vi "main-6003.vi"() -> ()   [LabVIEW 2018]
uses:
  <vilib>/Utility/miscctls.llb/LVPointDoubleTypeDef.ctl
  <vilib>/DAQmx/read.llb/DAQmx Read (Analog 1D Wfm NChan NSamp).vi
  <vilib>/Analysis/baseanly.llb/Mean (DBL).vi
  <vilib>/DAQmx/create/channels.llb/DAQmx Create Channel (AI-Voltage-Basic).vi
  <vilib>/DAQmx/configure/timing.llb/DAQmx Timing (Sample Clock).vi
  <vilib>/DAQmx/miscellaneous.llb/DAQmx Fill In Error Info.vi
  <vilib>/Waveform/WDTOps.llb/WDT Append Waveforms DBL.vi
  <vilib>/Utility/file.llb/Write To Spreadsheet File (DBL).vi
  <vilib>/Analysis/NI_AALBase.lvlib
  <resource>/objmgr/daqmx.rc
panel:
  out "当前":dbl
  in  "label":string
  out "时序":waveform(dbl)[](graph)
  out "判断类型":dbl
  out "可能性":dbl
  out "不同物品相似值":dbl[](graph)
  in  "?":bool
  in  "AIConv.Rate":dbl=5001.0
  in  "Channel":i32=1 min=1 max=6 step=1
  out "数组":string[](array[string])
  in  "选项卡控件":enum32{"Multichannel", "Single Channel"}(tab)
  out "Resistance":waveform(dbl)[](graph)
  out "Voltage":waveform(dbl)[](graph)
  in  "下拉列表 2":u16(ring) items=["Linear", "Log"]
  in  "Cursor":bool
  in  "下拉列表":u16(ring) items=["Linear", "Log"]
  in  "Cursor":bool
  out "游标.游标位置 2":T1 caption="游标.游标位置" {"Y" format="%#_5g"}
  out "游标.游标位置":T1
  out "游标.游标位置 4":T1 caption="游标.游标位置" {"Y" format="%#_5g"}
  in  "下拉列表 5":u16(ring) items=["Linear", "Log"]
  in  "Cursor":bool
  in  "下拉列表 4":u16(ring) items=["Linear", "Log"]
  in  "Cursor":bool
  out "Resistance":waveform(dbl)(graph)
  out "Voltage":waveform(dbl)(graph)
  out "游标.游标位置 3":T1 caption="游标.游标位置" {"Y" format="%#_5g"}
  out "元素 2":dbl format="%#_5g"
  out "元素":dbl format="%#_5p"
  in  "Resistance":dbl=100000.0
  in  "channel":i32=6 min=1 max=10 step=1
  in  "Voltage":dbl=1.0 min=-10.0 max=10.0
  out "default":path
  out "Elapsed Time (s)":dbl caption="Elapse Time"
  in  "确定按钮 2":bool
  in  "停止 2":bool
  in  "确定按钮":bool
  in  "停止":bool
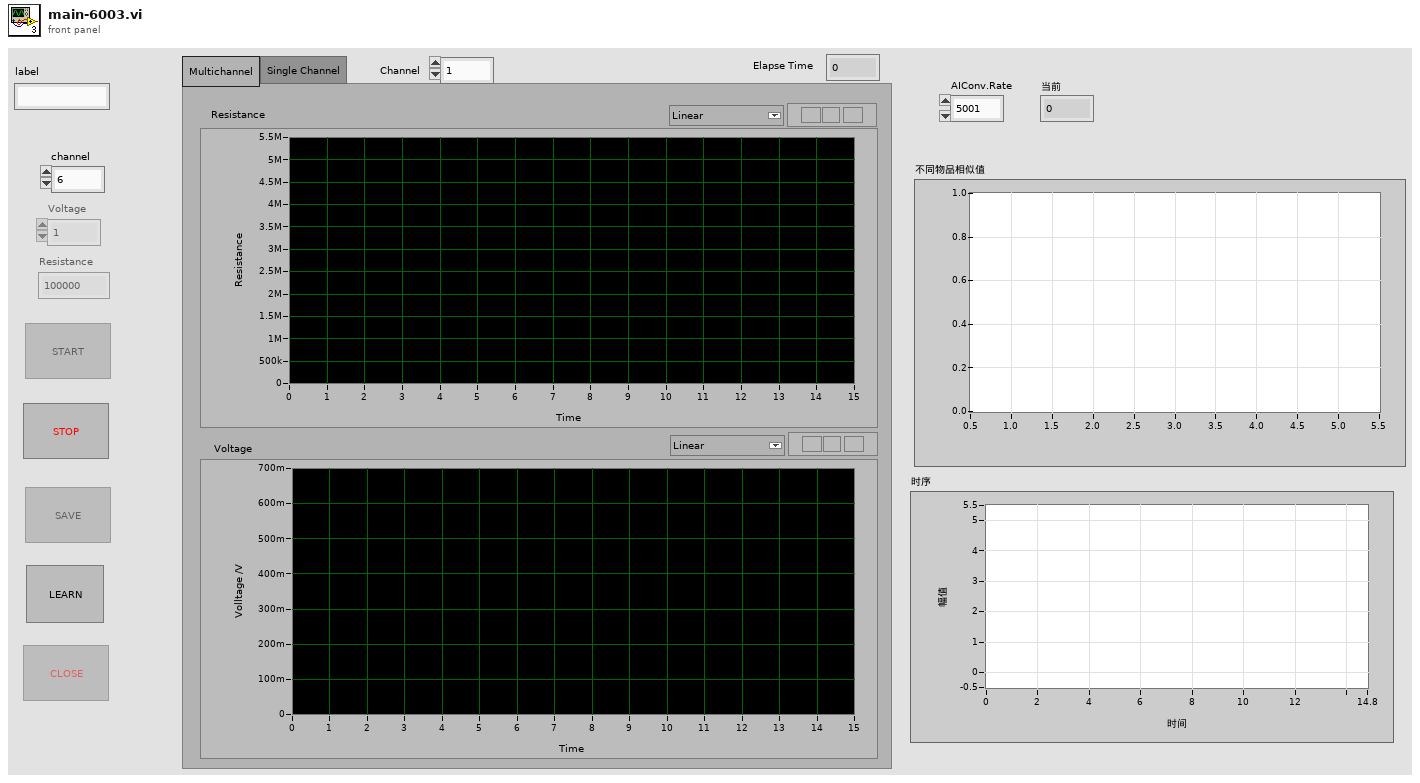
[diagram p1: front panel]
types:
  T1 = typedef "LVPointDoubleTypeDef.ctl" = cluster{"X":dbl, "Y":dbl}
  T2 = enum8{"Enabled", "Disabled", "Disabled and Grayed Out"}
  T3 = enum32{"invalid app kind", "Development System", "Run Time System", "Student Edition", "Embedded LabVIEW", "Evaluation", "Custom"}
  T4 = typedef "LVAnnotationListTypeDef.ctl" = cluster{"Name":string, "Color":u32, "Style":u8, "Point Style":u8, "Name Visible":bool, "Allow Drag":bool, "Annotation Mode":u32, "Plot":i32, "Index":i32, "Position":cluster{"X":dbl, "Y":dbl}, "X Scale":u32, "Y Scale":u32, "Show Arrow":bool, "Lock Name":bool, "Plot Area":i32, "Label Offset":cluster{"X":dbl, "Y":dbl}}[]
  T5 = cluster{"Name":string, "Color":u32, "Style":u8, "Point Style":u8, "Name Visible":bool, "Allow Drag":bool, "Annotation Mode":u32, "Plot":i32, "Index":i32, "Position":cluster{"X":dbl, "Y":dbl}, "X Scale":u32, "Y Scale":u32, "Show Arrow":bool, "Lock Name":bool, "Plot Area":i32, "Label Offset":cluster{"X":dbl, "Y":dbl}}
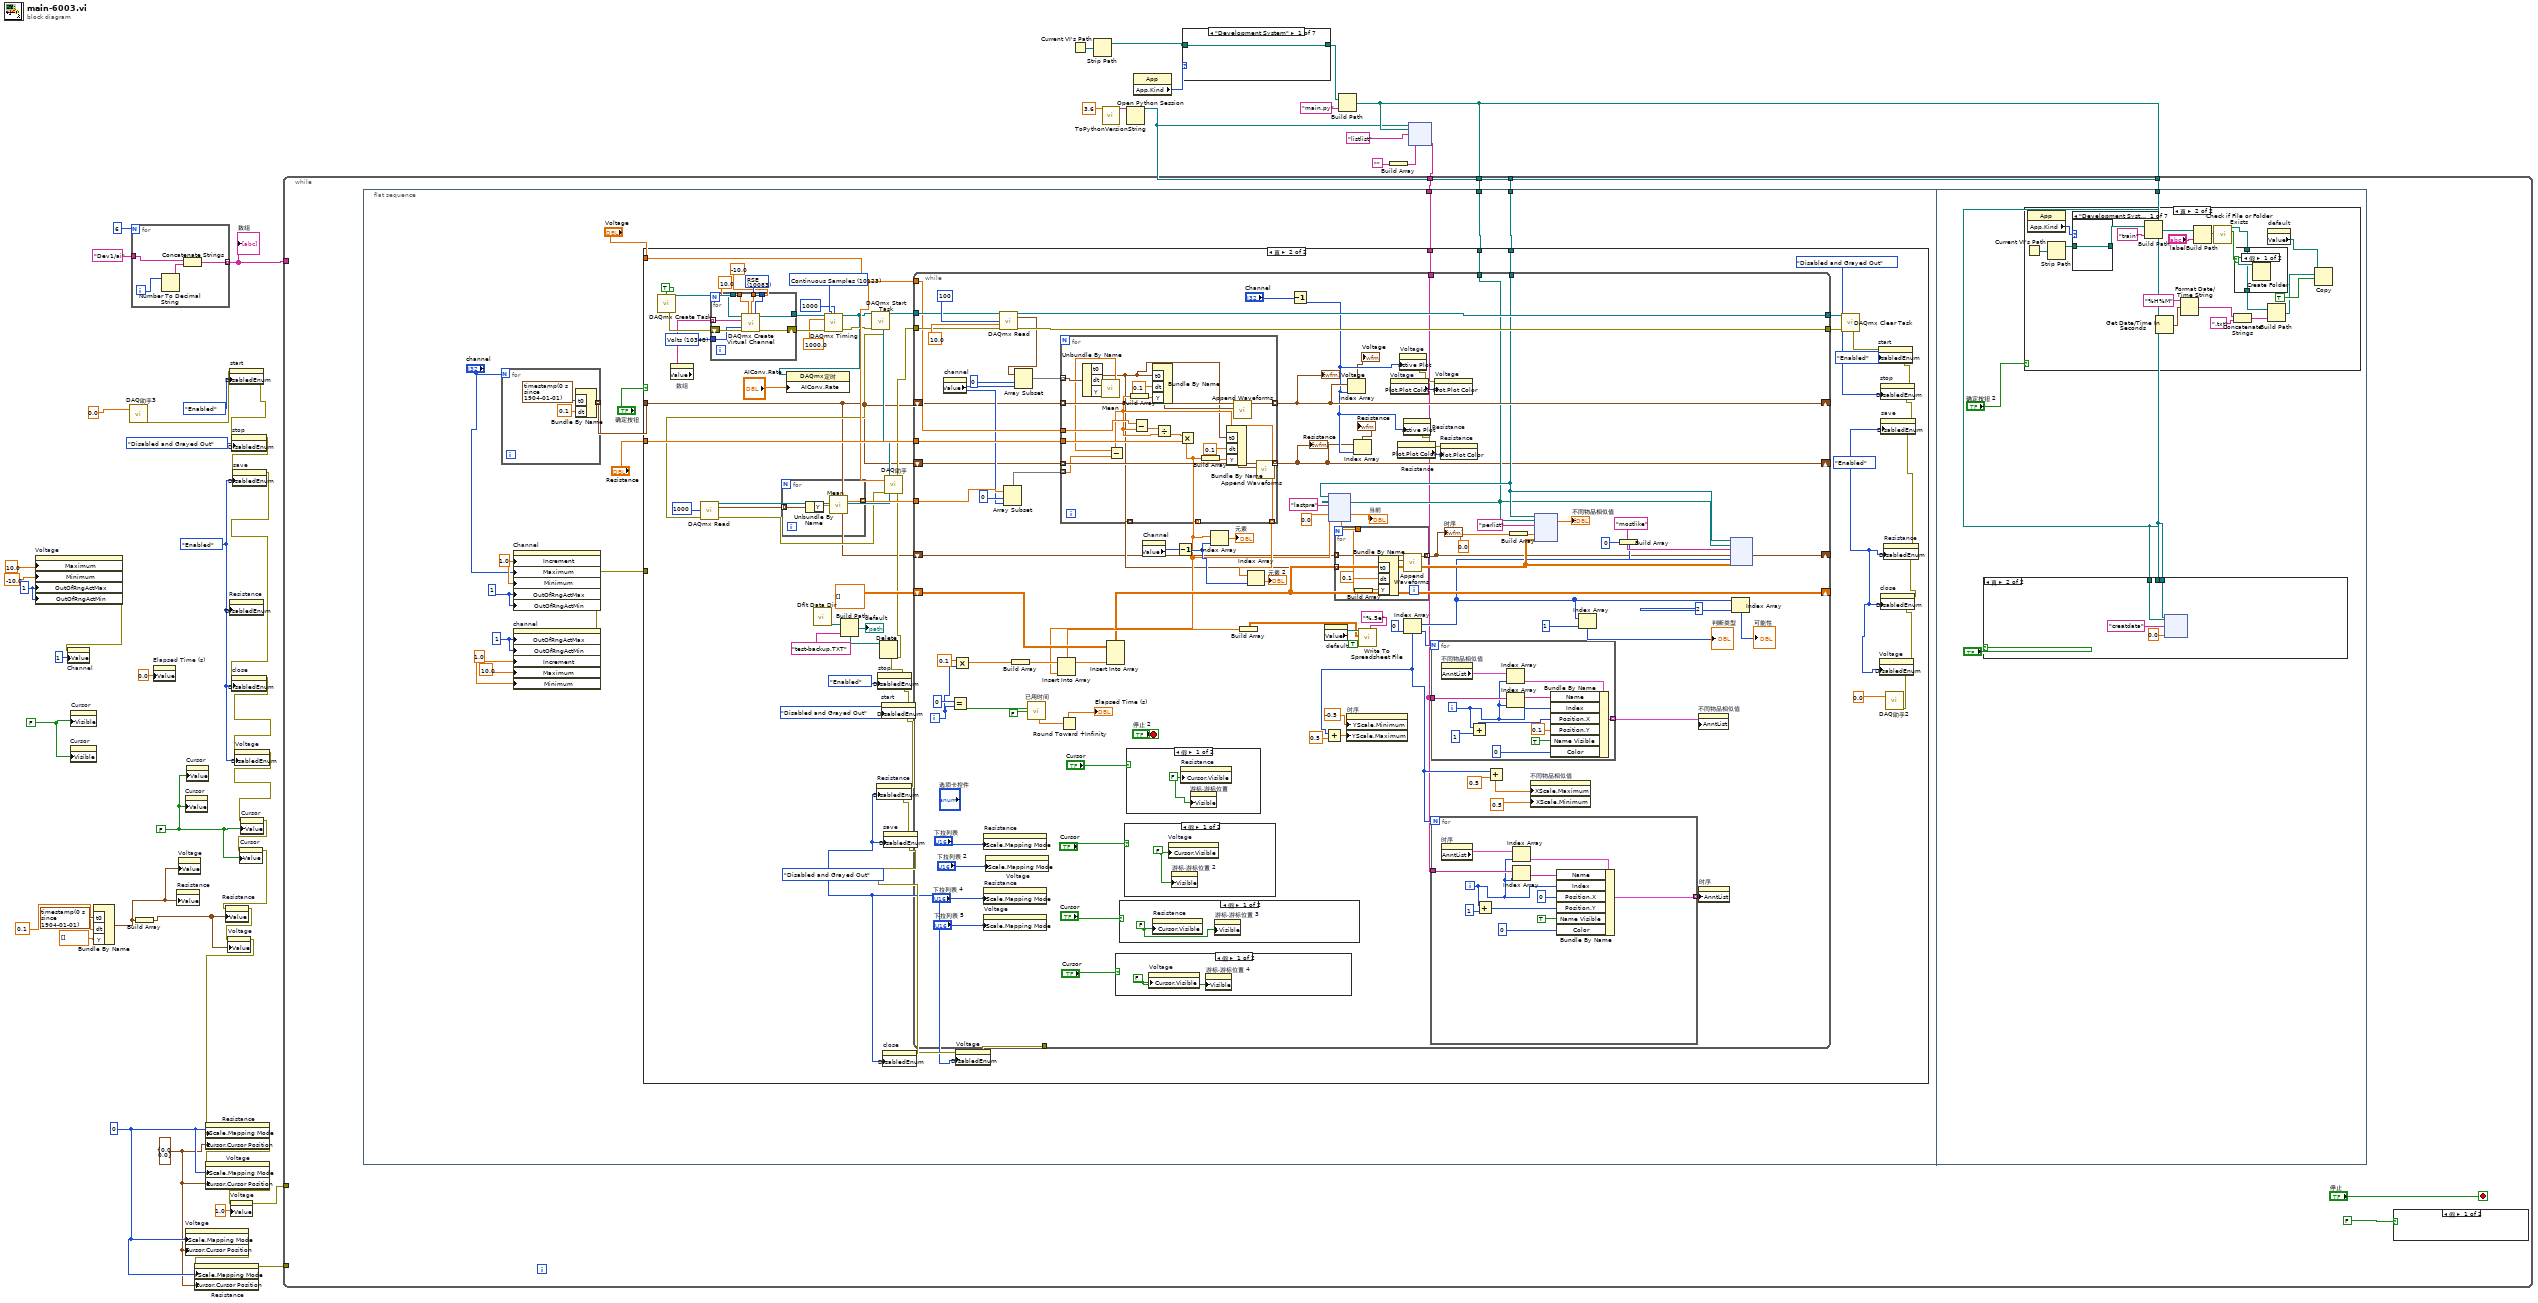
[diagram p0: block diagram]
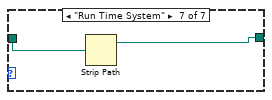
[diagram p7: hidden frame]
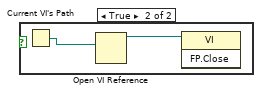
[diagram p8: hidden frame]
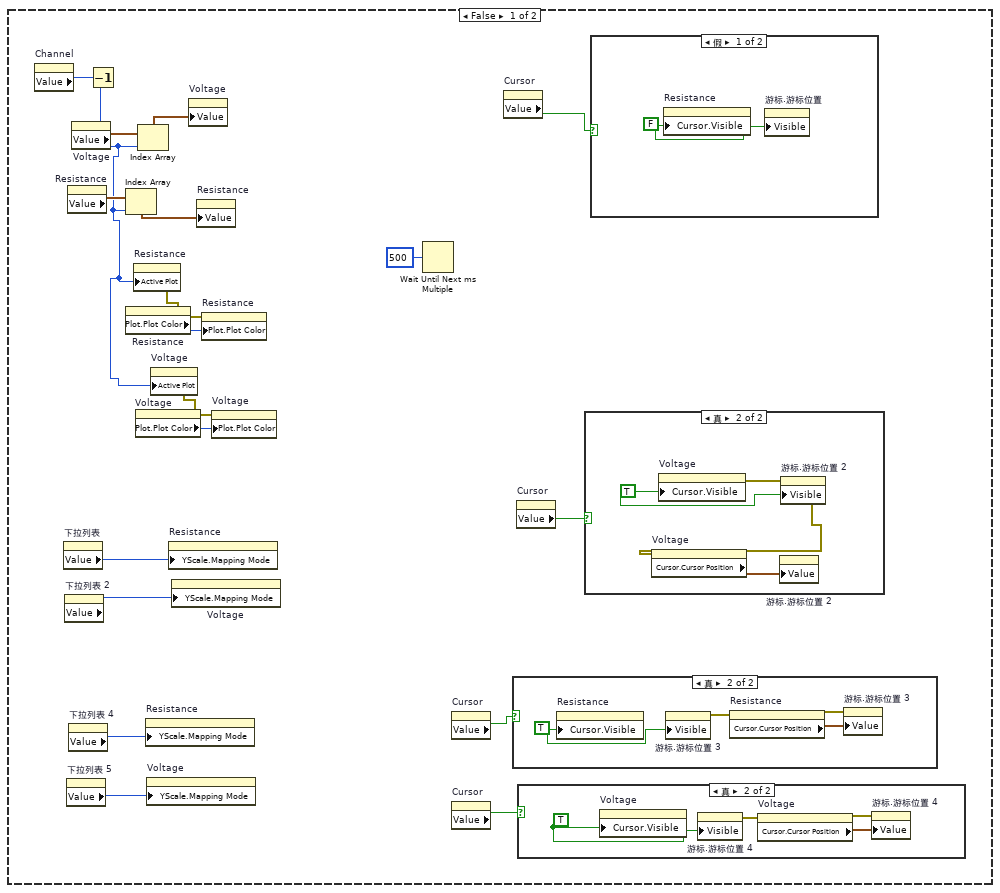
[diagram p9: hidden frame]
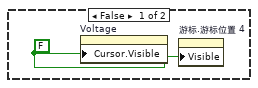
[diagram p10: hidden frame]
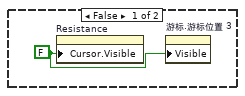
[diagram p11: hidden frame]
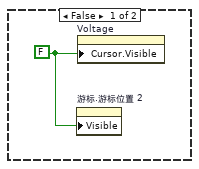
[diagram p12: hidden frame]
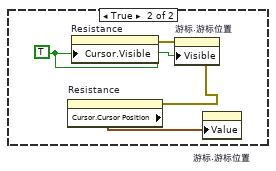
[diagram p13: hidden frame]
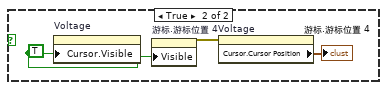
[diagram p14: hidden frame]
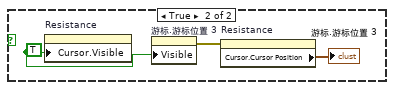
[diagram p15: hidden frame]
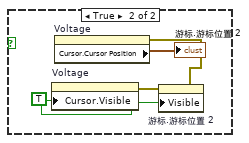
[diagram p16: hidden frame]
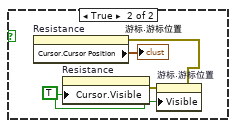
[diagram p17: hidden frame]
diagram:
  w19 = u8 1 ("对超出界限的值的响应:最大值")
  w28 = FALSE ("可见")
  w26 = FALSE ("Cursor")
  w24 = T1 {"X"=0.0, "Y"=0.0} ("游标.游标位置")
  w25 = u8 0 ("Y标尺.映射模式")
  w17 = T2."Enabled" ("禁用")
  n1 = property on="Voltage" class="DigNum (严格)"("Maximum"=10.0 ("数据输入界限:最大值"), "Minimum"=-10.0 ("数据输入界限:最大值"), "OutOfRngActMax"=w19, "OutOfRngActMin"=w19) -> (error out=w20:errorcluster)  [unwired: 2 in, 1 out]
  n2 = property on="Channel" class="DigNum (严格)"(error in=w20, "Value"=1 ("index (row)")) -> ()  [unwired: 1 in, 2 out]
  n3 = property on="Cursor" class="Bool (严格)"("Visible"=w28) -> ()  [unwired: 2 in, 2 out]
  n4 = property on="Cursor" class="Bool (严格)"("Visible"=w28) -> ()  [unwired: 2 in, 2 out]
  n5 = Bundle By Name("t0"=timestamp(0 s since 1904-01-01), "dt"=0.1, "Y"=dbl[] []) -> (w27:waveform(dbl))  [unwired: 1 in]
  n6 = call "DAQ助手3"("data"=0.0 ("maximum value")) -> ("error out"=w30:errorcluster)  [unwired: 17 in, 1 out]
  n7 = for {
    N: 6 -> [_]
    tunnel: "Dev1/ai" -> [w54]
    tunnel: [w52] -> w18 mode=indexing
    i -> [w55]
    n8 = Number To Decimal String(number=w55) -> (decimal integer string=w53:string)  [unwired: 1 in]
    n9 = Concatenate Strings(w54, w53) -> (w52:string)
  }
  "数组" <- w18
  n10 = Build Array(w27) -> (w32:waveform(dbl)[])
  n11 = property on="Elapsed Time (s)" class="DigNum (严格)"("Value"=0.0 ("Elapsed Time (s)")) -> ()  [unwired: 2 in, 2 out]
  n12 = property on="Resistance" class="WFGraph (严格)"("Value"=w27) -> ()  [unwired: 2 in, 2 out]
  n13 = property on="Voltage" class="WFGraph (严格)"("Value"=w27) -> ()  [unwired: 2 in, 2 out]
  n14 = property on="Cursor" class="Bool (严格)"("Value"=w26) -> ()  [unwired: 2 in, 2 out]
  n15 = property on="Voltage" class="WFGraph (严格)"("YScale.Mapping Mode"=w25, "Cursor.Cursor Position"=w24) -> (error out=w15:errorcluster)  [unwired: 2 in, 1 out]
  n16 = property on="Cursor" class="Bool (严格)"("Value"=w26) -> ()  [unwired: 2 in, 2 out]
  n17 = property on="Resistance" class="WFGraph (严格)"(error in=w15, "YScale.Mapping Mode"=w25, "Cursor.Cursor Position"=w24) -> (error out=w16:errorcluster)  [unwired: 1 in, 1 out]
  n18 = property on="Resistance" class="DigNum (严格)"("DisabledEnum"=w17) -> ()  [unwired: 2 in, 2 out]
  n19 = property on="start" class="Bool"(error in=w30, "DisabledEnum"=T2."Enabled" ("禁用")) -> (error out=w49:errorcluster)  [unwired: 1 in, 1 out]
  n20 = property on="stop" class="Bool"(error in=w49, "DisabledEnum"=T2."Disabled and Grayed Out" ("禁用")) -> (error out=w48:errorcluster)  [unwired: 1 in, 1 out]
  n21 = property on="save" class="Bool"(error in=w48, "DisabledEnum"=w17) -> (error out=w39:errorcluster)  [unwired: 1 in, 1 out]
  n22 = property on="close" class="Bool"(error in=w39, "DisabledEnum"=w17) -> (error out=w38:errorcluster)  [unwired: 1 in, 1 out]
  n23 = property on="Voltage" class="DigNum (严格)"(error in=w38, "DisabledEnum"=w17) -> (error out=w37:errorcluster)  [unwired: 1 in, 1 out]
  n24 = property on="Cursor" class="Bool (严格)"(error in=w37, "Value"=w26) -> (error out=w42:errorcluster)  [unwired: 1 in, 1 out]
  n25 = property on="Cursor" class="Bool (严格)"(error in=w42, "Value"=w26) -> (error out=w41:errorcluster)  [unwired: 1 in, 1 out]
  n26 = property on="Resistance" class="WFGraph (严格)"(error in=w41, "Value"=w32) -> (error out=w47:errorcluster)  [unwired: 1 in, 1 out]
  n27 = property on="Voltage" class="WFGraph (严格)"(error in=w47, "Value"=w32) -> (error out=w46:errorcluster)  [unwired: 1 in, 1 out]
  n28 = property on="Resistance" class="WFGraph (严格)"(error in=w46, "YScale.Mapping Mode"=w25, "Cursor.Cursor Position"=w24) -> (error out=w45:errorcluster)  [unwired: 1 in, 1 out]
  n29 = property on="Voltage" class="WFGraph (严格)"(error in=w45, "YScale.Mapping Mode"=w25, "Cursor.Cursor Position"=w24) -> (error out=w44:errorcluster)  [unwired: 1 in, 1 out]
  n30 = property on="Voltage" class="DigNum (严格)"(error in=w44, "Value"=1.0 ("Voltage")) -> (error out=w36:errorcluster)  [unwired: 1 in, 1 out]
  n31 = Current VI's Path() -> (path=w10:path)
  n32 = Strip Path(path=w10) -> (stripped path=w2:path)  [unwired: 1 out]
  n33 = call "ToPythonVersionString.vi"("Python版本"=3.6) -> ("python版本字符串"=w12:string)  [unwired: 10 in]
  n34 = Open Python Session(python version=w12) -> (session out=w4:refnum<k35>)  [unwired: 2 in, 1 out]
  n35 = property class="App"() -> ("App.Kind"=w3:T3)  [unwired: 2 in, 2 out]
  n36 = case shown="\"Development System\"" w3 {
    tunnel: w2 -> [w56 w57 w58 w59 w60 w61 w63]
    tunnel: [w56 w57 w58 w59 w60 w61 w62] -> w1
    frame "Development System" {
    }
    frame "Embedded LabVIEW" {
    }
    frame "Student Edition" {
    }
    frame "invalid app kind" {
    }
    frame "Custom" {
    }
    frame "Evaluation" {
    }
    frame "Run Time System" {
      n37 = Strip Path(path=w63) -> (stripped path=w62:path)  [unwired: 1 out]
    }
  }
  n38 = Build Path(base path=w1, name or relative path="main.py") -> (appended path=w5:path)
  n39 = Build Array("") -> (w7:string[])
  n40 = node(w4, w5, "listlist", w7) -> (w6:string[])  [unwired: 1 in, 4 out]
  n41 = while {
    tunnel: w36 -> [_]
    tunnel: w18 -> [_]
    tunnel: w16 -> [_]
    tunnel: w4 -> [w68]
    tunnel: w5 -> [w67]
    tunnel: w6 -> [w66]
    tunnel: w5 -> [w65]
    tunnel: w4 -> [w64]
    stop <- "停止" stop-if-true
    n42 = flat-sequence {
      tunnel: w66 -> [w75]
      tunnel: w65 -> [w74]
      tunnel: w64 -> [w73]
      tunnel: w68 -> [w360]
      tunnel: w67 -> [w359]
      frame #0 {
        w77 = 1.0 ("数据输入界限:增量")
        w78 = u8 1 ("对超出界限的值的响应:最小值")
        w81 = u8 1 ("对超出界限的值的响应:最小值")
        w83 = 1.0 ("数据输入界限:增量")
        n43 = for {
          N: "channel" -> [_]
          tunnel: [w88] -> w85 mode=indexing
          n44 = Bundle By Name("t0"=timestamp(0 s since 1904-01-01), "dt"=0.1) -> (w88:waveform(dbl))  [unwired: 1 in]
        }
        n45 = property on="Channel" class="DigNum (严格)"("Increment"=w83, "Maximum"="channel", "Minimum"=w83, "OutOfRngActMax"=w81, "OutOfRngActMin"=w81) -> (error out=w80:errorcluster)  [unwired: 2 in, 1 out]
        n46 = property on="channel" class="DigNum (严格)"(error in=w80, "OutOfRngActMax"=w78, "OutOfRngActMin"=w78, "Increment"=w77, "Maximum"=10.0 ("数据输入界限:增量"), "Minimum"=w77) -> (error out=w79:errorcluster)  [unwired: 1 in, 1 out]
        n47 = case shown="真" "确定按钮" {
          tunnel: "Voltage" -> [_ w170]
          tunnel: w85 -> [_ w133]
          tunnel: "Resistance" -> [_ w175]
          tunnel: w79 -> [_ _]
          tunnel: w75 -> [_ w132]
          tunnel: w74 -> [_ w135]
          tunnel: w73 -> [_ w134]
          frame False {
            n48 = property on="Channel" class="DigNum (严格)"() -> ("Value"=w98:i32)  [unwired: 2 in, 2 out]
            n49 = property on="下拉列表" class="Ring (严格)"() -> ("Value"=w109:u16)  [unwired: 2 in, 2 out]
            n50 = property on="下拉列表 2" class="Ring (严格)"() -> ("Value"=w110:u16)  [unwired: 2 in, 2 out]
            n51 = property on="下拉列表 5" class="Ring (严格)"() -> ("Value"=w106:u16)  [unwired: 2 in, 2 out]
            n52 = property on="Resistance" class="WFGraph (严格)"() -> ("Value"=w101:waveform(dbl)[])  [unwired: 2 in, 2 out]
            n53 = property on="下拉列表 4" class="Ring (严格)"() -> ("Value"=w105:u16)  [unwired: 2 in, 2 out]
            n54 = property on="Voltage" class="WFGraph (严格)"() -> ("Value"=w99:waveform(dbl)[])  [unwired: 2 in, 2 out]
            n55 = Decrement(x=w98) -> (x-1=w92:i32)
            n56 = Index Array(array=w101, index=w92) -> (element=w102:waveform(dbl))
            n57 = property on="Resistance" class="WFGraph (严格)"("Active Plot"=w92) -> (error out=w97:errorcluster)  [unwired: 2 in, 1 out]
            n58 = property on="Resistance" class="WFGraph (严格)"(error in=w97) -> (error out=w95:errorcluster, "Plot.Plot Color"=w96:u32)  [unwired: 1 in, 1 out]
            n59 = Index Array(array=w99, index=w92) -> (element=w100:waveform(dbl))
            n60 = property on="Resistance" class="WFGraph (严格)"("YScale.Mapping Mode"=w105) -> ()  [unwired: 2 in, 2 out]
            n61 = property on="Voltage" class="WFGraph (严格)"("YScale.Mapping Mode"=w106) -> ()  [unwired: 2 in, 2 out]
            n62 = property on="Voltage" class="WFGraph (严格)"("Active Plot"=w92) -> (error out=w91:errorcluster)  [unwired: 2 in, 1 out]
            n63 = property on="Voltage" class="WFGraph (严格)"(error in=w91) -> (error out=w94:errorcluster, "Plot.Plot Color"=w93:u32)  [unwired: 1 in, 1 out]
            n64 = property on="Resistance" class="WFGraph (严格)"("YScale.Mapping Mode"=w109) -> ()  [unwired: 2 in, 2 out]
            n65 = property on="Voltage" class="WFGraph (严格)"("YScale.Mapping Mode"=w110) -> ()  [unwired: 2 in, 2 out]
            n66 = property on="Voltage" class="WFGraph (严格)"("Value"=w100) -> ()  [unwired: 2 in, 2 out]
            n67 = property on="Resistance" class="WFGraph (严格)"("Value"=w102) -> ()  [unwired: 2 in, 2 out]
            n68 = property on="Resistance" class="WFGraph (严格)"(error in=w95, "Plot.Plot Color"=w96) -> ()  [unwired: 1 in, 2 out]
            n69 = property on="Voltage" class="WFGraph (严格)"(error in=w94, "Plot.Plot Color"=w93) -> ()  [unwired: 1 in, 2 out]
            n70 = Wait Until Next ms Multiple(millisecond multiple=u32 500 ("毫秒倍数")) -> ()  [unwired: 1 out]
            n71 = property on="Cursor" class="Bool (严格)"() -> ("Value"=w103:bool)  [unwired: 2 in, 2 out]
            n72 = property on="Cursor" class="Bool (严格)"() -> ("Value"=w104:bool)  [unwired: 2 in, 2 out]
            n73 = property on="Cursor" class="Bool (严格)"() -> ("Value"=w108:bool)  [unwired: 2 in, 2 out]
            n74 = case shown="真" w103 {
              frame False {
                w117 = FALSE ("游标.可见")
                n75 = property on="Resistance" class="WFGraph (严格)"("Cursor.Visible"=w117) -> ()  [unwired: 2 in, 2 out]
                n76 = property on="游标.游标位置 3" class="Clust (严格)"("Visible"=w117) -> ()  [unwired: 2 in, 2 out]
              }
              frame True {
                w121 = TRUE ("游标.可见")
                n77 = property on="Resistance" class="WFGraph (严格)"("Cursor.Visible"=w121) -> ()  [unwired: 2 in, 2 out]
                n78 = property on="游标.游标位置 3" class="Clust (严格)"("Visible"=w121) -> (error out=w120:errorcluster)  [unwired: 2 in, 1 out]
                n79 = property on="Resistance" class="WFGraph (严格)"(error in=w120) -> (error out=w119:errorcluster, "Cursor.Cursor Position"=w118:T1)  [unwired: 1 in, 1 out]
                n80 = property on="游标.游标位置 3" class="Clust (严格)"(error in=w119, "Value"=w118) -> ()  [unwired: 1 in, 2 out]
              }
            }
            n81 = property on="Cursor" class="Bool (严格)"() -> ("Value"=w107:bool)  [unwired: 2 in, 2 out]
            n82 = case shown="真" w104 {
              frame False {
                w112 = FALSE ("游标.可见")
                n83 = property on="Voltage" class="WFGraph (严格)"("Cursor.Visible"=w112) -> ()  [unwired: 2 in, 2 out]
                n84 = property on="游标.游标位置 4" class="Clust (严格)"("Visible"=w112) -> ()  [unwired: 2 in, 2 out]
              }
              frame True {
                w116 = TRUE ("游标.可见")
                n85 = property on="Voltage" class="WFGraph (严格)"("Cursor.Visible"=w116) -> ()  [unwired: 2 in, 2 out]
                n86 = property on="游标.游标位置 4" class="Clust (严格)"("Visible"=w116) -> (error out=w115:errorcluster)  [unwired: 2 in, 1 out]
                n87 = property on="Voltage" class="WFGraph (严格)"(error in=w115) -> (error out=w114:errorcluster, "Cursor.Cursor Position"=w113:T1)  [unwired: 1 in, 1 out]
                n88 = property on="游标.游标位置 4" class="Clust (严格)"(error in=w114, "Value"=w113) -> ()  [unwired: 1 in, 2 out]
              }
            }
            n89 = case shown="真" w107 {
              frame False {
                w122 = FALSE ("游标.可见")
                n90 = property on="游标.游标位置 2" class="Clust (严格)"("Visible"=w122) -> ()  [unwired: 2 in, 2 out]
                n91 = property on="Voltage" class="WFGraph (严格)"("Cursor.Visible"=w122) -> ()  [unwired: 2 in, 2 out]
              }
              frame True {
                w126 = TRUE ("游标.可见")
                n92 = property on="Voltage" class="WFGraph (严格)"("Cursor.Visible"=w126) -> (error out=w125:errorcluster)  [unwired: 2 in, 1 out]
                n93 = property on="游标.游标位置 2" class="Clust (严格)"(error in=w125, "Visible"=w126) -> (error out=w123:errorcluster)  [unwired: 1 in, 1 out]
                n94 = property on="Voltage" class="WFGraph (严格)"(error in=w123) -> ("Cursor.Cursor Position"=w124:T1)  [unwired: 1 in, 2 out]
                n95 = property on="游标.游标位置 2" class="Clust (严格)"("Value"=w124) -> ()  [unwired: 2 in, 2 out]
              }
            }
            n96 = case shown="假" w108 {
              frame False {
                w127 = FALSE ("游标.可见")
                n97 = property on="Resistance" class="WFGraph (严格)"("Cursor.Visible"=w127) -> ()  [unwired: 2 in, 2 out]
                n98 = property on="游标.游标位置" class="Clust (严格)"("Visible"=w127) -> ()  [unwired: 2 in, 2 out]
              }
              frame True {
                w131 = TRUE ("游标.可见")
                n99 = property on="Resistance" class="WFGraph (严格)"("Cursor.Visible"=w131) -> (error out=w130:errorcluster)  [unwired: 2 in, 1 out]
                n100 = property on="游标.游标位置" class="Clust (严格)"(error in=w130, "Visible"=w131) -> (error out=w129:errorcluster)  [unwired: 1 in, 1 out]
                n101 = property on="Resistance" class="WFGraph (严格)"(error in=w129) -> ("Cursor.Cursor Position"=w128:T1)  [unwired: 1 in, 2 out]
                n102 = property on="游标.游标位置" class="Clust (严格)"("Value"=w128) -> ()  [unwired: 2 in, 2 out]
              }
            }
          }
          frame True {
            w161 = 10123 items=["Finite Samples"=10178, "Continuous Samples"=10123, "Hardware Timed Single Point"=12522] ("sample mode")
            w157 = 10348 items=["Volts"=10348, "From Custom Scale"=10065] ("units")
            w156 = 10083 items=["default"=-1, "RSE"=10083, "NRSE"=10078, "Differential"=10106, "Pseudodifferential"=12529] ("input terminal configuration")
            w149 = T2."Enabled" ("禁用")
            w150 = T2."Disabled and Grayed Out" ("禁用")
            n103 = call <vilib>:"DAQmx Create Task.vi"("auto cleanup"=TRUE) -> ("task out"=w158:refnum<k21>, "error out"=w159:errorcluster)  [unwired: 13 in]
            n104 = property on="数组" class="Arr (严格)"() -> ("Value"=w152:string[])  [unwired: 2 in, 2 out]
            n105 = for {
              tunnel: [w199] -> w163
              tunnel: w158 -> [w198]
              tunnel: 10.0 ("maximum value") -> [w197]
              tunnel: -10.0 ("maximum value") -> [w196]
              shift-right: [w194] -> w164
              shift-left: w159 -> [w195]
              tunnel: w156 -> [w193]
              tunnel: w152 -> [w192] mode=indexing
              tunnel: w157 -> [w191]
              n106 = call-poly <vilib>:"DAQmx Create Virtual Channel.vi"("task in"=w198, "maximum value"=w197, "minimum value"=w196, "input terminal configuration"=w193, "physical channels"=w192, "units"=w191, "error in"=w195) -> ("task out"=w199:refnum<k21>, "error out"=w194:errorcluster)  [unwired: 7 in]
            }
            n107 = call <vilib>:"Dflt Data Dir.vi"() -> ("App:Default Data Directory"=w186:path)
            n108 = call-poly <vilib>:"DAQmx Timing.vi"("task/channels in"=w163, "sample mode"=w161, "samples per channel"=1000, "rate"=1000.0, "error in"=w164) -> ("task out"=w137:refnum<k21>, "error out"=w151:errorcluster)  [unwired: 9 in]
            n109 = property class="DAQmx定时"(reference=w137, "AIConv.Rate"="AIConv.Rate") -> ()  [unwired: 1 in, 2 out]
            n110 = Build Path(base path=w186, name or relative path="test-backup.TXT" ("名称或相对路径")) -> (appended path=w184:path)
            "default" <- w184
            n111 = call <vilib>:"DAQmx Start Task.vi"("task/channels in"=w137, "error in"=w151) -> ("task out"=w143:refnum<k21>, "error out"=w141:errorcluster)  [unwired: 12 in]
            n112 = call-poly <vilib>:"DAQmx Read.vi"("task/channels in"=w143, "number of samples per channel"=1000, "error in"=w141) -> ("data"=w139:waveform(dbl)[], "error out"=w142:errorcluster)  [unwired: 10 in, 1 out]
            n113 = for {
              tunnel: w139 -> [w190] mode=indexing
              tunnel: [w188] -> w144 mode=indexing
              n114 = Unbundle By Name(w190) -> ("Y"=w189:dbl[])
              n115 = call-poly <vilib>:"Mean.vi"("X"=w189) -> ("mean"=w188:dbl)  [unwired: 1 out]
            }
            n116 = call "DAQ助手"("data"=w170, "error in"=w142) -> ("error out"=w140:errorcluster)  [unwired: 16 in, 1 out]
            n117 = Delete(path (use dialog)=w184, error in=w140) -> (error out=w182:errorcluster)  [unwired: 3 in, 2 out]
            n118 = property on="stop" class="Bool"(error in=w182, "DisabledEnum"=T2."Enabled" ("禁用")) -> (error out=w180:errorcluster)  [unwired: 1 in, 1 out]
            n119 = property on="start" class="Bool"(error in=w180, "DisabledEnum"=T2."Disabled and Grayed Out" ("禁用")) -> (error out=w148:errorcluster)  [unwired: 1 in, 1 out]
            n120 = property on="Resistance" class="DigNum (严格)"(error in=w148, "DisabledEnum"=w150) -> (error out=w147:errorcluster)  [unwired: 1 in, 1 out]
            n121 = property on="save" class="Bool"(error in=w147, "DisabledEnum"=w150) -> (error out=w174:errorcluster)  [unwired: 1 in, 1 out]
            n122 = property on="close" class="Bool"(error in=w174, "DisabledEnum"=w150) -> (error out=w173:errorcluster)  [unwired: 1 in, 1 out]
            n123 = property on="Voltage" class="DigNum (严格)"(error in=w173, "DisabledEnum"=w150) -> (error out=w172:errorcluster)  [unwired: 1 in, 1 out]
            n124 = while {
              tunnel: [w273] -> w167
              tunnel: [w272] -> w166
              tunnel: w170 -> [w271]
              shift-right: [w228] -> _
              shift-left: dbl[][] [] -> [w265]
              tunnel: w172 -> [_]
              tunnel: w143 -> [w275]
              tunnel: w140 -> [w274]
              tunnel: w175 -> [w270]
              shift-right: [w263] -> _
              shift-left: w133 -> [w210]
              shift-right: [w205] -> _
              shift-left: w133 -> [w212]
              tunnel: w144 -> [w240]
              tunnel: w135 -> [w226]
              tunnel: w134 -> [w227]
              shift-right: [w208] -> _
              shift-left: w133 -> [w209]
              tunnel: w132 -> [w201]
              i -> [w268]
              stop <- "停止 2" stop-if-true
              n125 = property on="channel" class="DigNum (严格)"() -> ("Value"=w238:i32)  [unwired: 2 in, 2 out]
              n126 = Equal?(x=0, y=w268) -> (x = y?=w283:bool)
              n127 = Multiply(x=0.1, y=w268) -> (x*y=w267:dbl)
              n128 = property on="Resistance" class="WFGraph (严格)"("YScale.Mapping Mode"="下拉列表") -> ()  [unwired: 2 in, 2 out]
              n129 = property on="Resistance" class="WFGraph (严格)"("YScale.Mapping Mode"="下拉列表 4") -> ()  [unwired: 2 in, 2 out]
              n130 = property on="Voltage" class="WFGraph (严格)"("YScale.Mapping Mode"="下拉列表 5") -> ()  [unwired: 2 in, 2 out]
              n131 = property on="Voltage" class="WFGraph (严格)"("YScale.Mapping Mode"="下拉列表 2") -> ()  [unwired: 2 in, 2 out]
              n132 = call-poly <vilib>:"DAQmx Read.vi"("task/channels in"=w275, "number of samples per channel"=100, "timeout"=10.0, "error in"=w274) -> ("task out"=w273:refnum<k21>, "data"=w236:waveform(dbl)[], "error out"=w272:errorcluster)  [unwired: 9 in]
              n133 = Array Subset(array=w240, index=0 ("索引"), length=w238) -> (w237:dbl[])
              n134 = Build Array(w267) -> (w266:dbl[])
              n135 = Array Subset(array=w236, index=0 ("索引"), length=w238) -> (w259:waveform(dbl)[])
              n136 = call "已用时间"("Reset"=w283, "Auto Reset"=FALSE) -> ("Elapsed Time (s)"=w280:dbl)  [unwired: 10 in, 7 out]
              n137 = Round Toward +Infinity(x=w280) -> (ceil(x): smallest int >= x=→"Elapsed Time (s)":dbl)
              n138 = for {
                tunnel: w259 -> [w348] mode=indexing
                tunnel: w210 -> [w343] mode=indexing
                tunnel: [w347] -> w263 mode=indexing
                tunnel: w271 -> [w341]
                tunnel: w270 -> [w338]
                tunnel: [w334] -> w205 mode=indexing
                tunnel: w212 -> [w333] mode=indexing
                tunnel: [w329] -> w213 mode=indexing
                tunnel: [w330] -> w244 mode=indexing
                tunnel: w237 -> [w331] mode=indexing
                tunnel: [w328] -> w211 mode=indexing
                n139 = Unbundle By Name(w348) -> ("t0"=w328:timestamp, "Y"=w346:dbl[])  [unwired: 1 out]
                n140 = call-poly <vilib>:"Mean.vi"("X"=w346) -> ("mean"=w332:dbl)  [unwired: 1 out]
                n141 = Subtract(x=w332, y=w331) -> (x-y=w330:dbl)
                n142 = Build Array(w330) -> (w345:dbl[])
                n143 = Subtract(x=w341, y=w330) -> (x-y=w340:dbl)
                n144 = Bundle By Name("t0"=w328, "dt"=0.1, "Y"=w345) -> (w342:waveform(dbl))  [unwired: 1 in]
                n145 = Divide(x=w340, y=w330) -> (x/y=w339:dbl)
                n146 = Multiply(x=w339, y=w338) -> (x*y=w329:dbl)
                n147 = Build Array(w329) -> (w336:dbl[])
                n148 = Bundle By Name("t0"=w328, "dt"=0.1, "Y"=w336) -> (w335:waveform(dbl))  [unwired: 1 in]
                n149 = call-poly <vilib>:"Append Waveforms.vi"("waveform B"=w342, "waveform A"=w343) -> ("waveform out"=w347:waveform(dbl))  [unwired: 8 in, 1 out]
                n150 = call-poly <vilib>:"Append Waveforms.vi"("waveform B"=w335, "waveform A"=w333) -> ("waveform out"=w334:waveform(dbl))  [unwired: 8 in, 1 out]
              }
              "Voltage" <- w263
              "Resistance" <- w205
              n151 = Insert Into Array(array=w266, new element=w213) -> (w261:dbl[])  [unwired: 1 in]
              n152 = Insert Into Array(array=w265, new element=w261) -> (w228:dbl[][])  [unwired: 2 in]
              n153 = case shown="假" "Cursor" {
                frame False {
                  w320 = FALSE ("游标.可见")
                  n154 = property on="Voltage" class="WFGraph (严格)"("Cursor.Visible"=w320) -> ()  [unwired: 2 in, 2 out]
                  n155 = property on="游标.游标位置 4" class="Clust (严格)"("Visible"=w320) -> ()  [unwired: 2 in, 2 out]
                }
                frame True {
                  w323 = TRUE ("游标.可见")
                  n156 = property on="Voltage" class="WFGraph (严格)"("Cursor.Visible"=w323) -> ()  [unwired: 2 in, 2 out]
                  n157 = property on="游标.游标位置 4" class="Clust (严格)"("Visible"=w323) -> (error out=w322:errorcluster)  [unwired: 2 in, 1 out]
                  n158 = property on="Voltage" class="WFGraph (严格)"(error in=w322) -> ("Cursor.Cursor Position"=→"游标.游标位置 4":T1)  [unwired: 1 in, 2 out]
                }
              }
              n159 = case shown="假" "Cursor" {
                frame False {
                  w324 = FALSE ("游标.可见")
                  n160 = property on="Resistance" class="WFGraph (严格)"("Cursor.Visible"=w324) -> ()  [unwired: 2 in, 2 out]
                  n161 = property on="游标.游标位置 3" class="Clust (严格)"("Visible"=w324) -> ()  [unwired: 2 in, 2 out]
                }
                frame True {
                  w327 = TRUE ("游标.可见")
                  n162 = property on="Resistance" class="WFGraph (严格)"("Cursor.Visible"=w327) -> ()  [unwired: 2 in, 2 out]
                  n163 = property on="游标.游标位置 3" class="Clust (严格)"("Visible"=w327) -> (error out=w326:errorcluster)  [unwired: 2 in, 1 out]
                  n164 = property on="Resistance" class="WFGraph (严格)"(error in=w326) -> ("Cursor.Cursor Position"=→"游标.游标位置 3":T1)  [unwired: 1 in, 2 out]
                }
              }
              n165 = case shown="假" "Cursor" {
                frame False {
                  w349 = FALSE ("游标.可见")
                  n166 = property on="Voltage" class="WFGraph (严格)"("Cursor.Visible"=w349) -> ()  [unwired: 2 in, 2 out]
                  n167 = property on="游标.游标位置 2" class="Clust (严格)"("Visible"=w349) -> ()  [unwired: 2 in, 2 out]
                }
                frame True {
                  w352 = TRUE ("游标.可见")
                  n168 = property on="Voltage" class="WFGraph (严格)"("Cursor.Visible"=w352) -> (error out=w351:errorcluster)  [unwired: 2 in, 1 out]
                  n169 = property on="游标.游标位置 2" class="Clust (严格)"(error in=w351, "Visible"=w352) -> (error out=w350:errorcluster)  [unwired: 1 in, 1 out]
                  n170 = property on="Voltage" class="WFGraph (严格)"(error in=w350) -> ("Cursor.Cursor Position"=→"游标.游标位置 2":T1)  [unwired: 1 in, 2 out]
                }
              }
              n171 = case shown="假" "Cursor" {
                frame False {
                  w354 = FALSE ("游标.可见")
                  n172 = property on="Resistance" class="WFGraph (严格)"("Cursor.Visible"=w354) -> ()  [unwired: 2 in, 2 out]
                  n173 = property on="游标.游标位置" class="Clust (严格)"("Visible"=w354) -> ()  [unwired: 2 in, 2 out]
                }
                frame True {
                  w357 = TRUE ("游标.可见")
                  n174 = property on="Resistance" class="WFGraph (严格)"("Cursor.Visible"=w357) -> (error out=w356:errorcluster)  [unwired: 2 in, 1 out]
                  n175 = property on="游标.游标位置" class="Clust (严格)"(error in=w356, "Visible"=w357) -> (error out=w355:errorcluster)  [unwired: 1 in, 1 out]
                  n176 = property on="Resistance" class="WFGraph (严格)"(error in=w355) -> ("Cursor.Cursor Position"=→"游标.游标位置":T1)  [unwired: 1 in, 2 out]
                }
              }
              n177 = property on="Channel" class="DigNum (严格)"() -> ("Value"=w242:i32)  [unwired: 2 in, 2 out]
              n178 = Decrement(x=w242) -> (x-1=w241:i32)
              n179 = Index Array(array=w213, index=w241) -> (element=→"元素":dbl)
              n180 = Build Array(w261) -> (w262:dbl[][])
              n181 = Index Array(array=w244, index=w241) -> (element=→"元素 2":dbl)
              n182 = Decrement(x="Channel") -> (x-1=w251:i32)
              n183 = property on="default" class="Path"() -> ("Value"=w278:path)  [unwired: 2 in, 2 out]
              n184 = node(w227, w226, "lastpre", 0.0, w213) -> (w200:dbl)  [unwired: 2 in, 4 out]
              "当前" <- w200
              n185 = for {
                tunnel: w200 -> [w306]
                tunnel: [w304] -> w208 mode=indexing
                tunnel: w211 -> [w303] mode=indexing
                tunnel: w209 -> [w302] mode=indexing
                n186 = Build Array(w306) -> (w305:dbl[])
                n187 = Bundle By Name("t0"=w303, "dt"=0.1, "Y"=w305) -> (w308:waveform(dbl))  [unwired: 1 in]
                n188 = call-poly <vilib>:"Append Waveforms.vi"("waveform B"=w308, "waveform A"=w302) -> ("waveform out"=w304:waveform(dbl))  [unwired: 8 in, 1 out]
              }
              "时序" <- w208
              n189 = Index Array(array=w263, index=w251) -> (element=→"Voltage":waveform(dbl))
              n190 = Index Array(array=w205, index=w251) -> (element=→"Resistance":waveform(dbl))
              n191 = call-poly <vilib>:"Write To Spreadsheet File.vi"("format (%.3f)"="%.5e", "append to file? (new file:F)"=TRUE, "2D data"=w262, "file path (dialog if empty)"=w278) -> ()  [unwired: 4 in, 1 out]
              n192 = property on="Voltage" class="WFGraph (严格)"("Active Plot"=w251) -> (error out=w250:errorcluster)  [unwired: 2 in, 1 out]
              n193 = property on="Voltage" class="WFGraph (严格)"(error in=w250) -> (error out=w249:errorcluster, "Plot.Plot Color"=w248:u32)  [unwired: 1 in, 1 out]
              n194 = property on="Resistance" class="WFGraph (严格)"("Active Plot"=w251) -> (error out=w252:errorcluster)  [unwired: 2 in, 1 out]
              n195 = property on="Resistance" class="WFGraph (严格)"(error in=w252) -> (error out=w254:errorcluster, "Plot.Plot Color"=w253:u32)  [unwired: 1 in, 1 out]
              n196 = property on="Voltage" class="WFGraph (严格)"(error in=w249, "Plot.Plot Color"=w248) -> ()  [unwired: 1 in, 2 out]
              n197 = property on="Resistance" class="WFGraph (严格)"(error in=w254, "Plot.Plot Color"=w253) -> ()  [unwired: 1 in, 2 out]
              n198 = Build Array(0.0) -> (w232:dbl[])
              n199 = node(w227, w226, "perlist", w232, w228) -> (→"不同物品相似值":dbl[])  [unwired: 2 in, 4 out]
              n200 = Build Array(0) -> (w223:i32[])
              n201 = node(w227, w226, "mostlike", w223, w228) -> (w219:i32[])  [unwired: 2 in, 4 out]
              n202 = Index Array(array=w219, index=0) -> (element=w204:i32)
              n203 = Add(x=w204, y=0.5) -> (x+y=w202:dbl)
              n204 = property on="时序" class="WFGraph (严格)"("YScale.Minimum"=-0.5, "YScale.Maximum"=w202) -> ()  [unwired: 2 in, 2 out]
              n205 = for {
                N: w204 -> [_]
                tunnel: [w318] -> w235 mode=indexing
                tunnel: w201 -> [w315]
                i -> [w310]
                n206 = property on="不同物品相似值" class="WFGraph (严格)"() -> ("AnntList"=w313:T4)  [unwired: 2 in, 2 out]
                n207 = Add(x=w310, y=1) -> (x+y=w309:i32)
                n208 = Index Array(array=w313, index=w310) -> (element=w319:T5)
                n209 = Index Array(array=w315, index=w310) -> (element=w314:string)
                n210 = Bundle By Name(cluster=w319, "Name"=w314, "Index"=w310, "Position.X"=w309, "Position.Y"=0.1, "Name Visible"=TRUE, "Color"=0) -> (w318:T5)
              }
              n211 = for {
                N: w204 -> [_]
                tunnel: [w300] -> w206 mode=indexing
                tunnel: w201 -> [w295]
                i -> [w294]
                n212 = property on="时序" class="WFGraph (严格)"() -> ("AnntList"=w296:T4)  [unwired: 2 in, 2 out]
                n213 = Add(x=w294, y=1) -> (x+y=w292:i32)
                n214 = Index Array(array=w296, index=w294) -> (element=w301:T5)
                n215 = Index Array(array=w295, index=w294) -> (element=w293:string)
                n216 = Bundle By Name(cluster=w301, "Name"=w293, "Index"=w294, "Position.X"=0, "Position.Y"=w292, "Name Visible"=TRUE, "Color"=0) -> (w300:T5)
              }
              n217 = Add(x=w204, y=0.5) -> (x+y=w215:dbl)
              n218 = property on="不同物品相似值" class="WFGraph (严格)"("XScale.Maximum"=w215, "XScale.Minimum"=0.5) -> ()  [unwired: 2 in, 2 out]
              n219 = Index Array(array=w219, index=1) -> (element=→"判断类型":i32)
              n220 = property on="不同物品相似值" class="WFGraph (严格)"("AnntList"=w235) -> ()  [unwired: 2 in, 2 out]
              n221 = property on="时序" class="WFGraph (严格)"("AnntList"=w206) -> ()  [unwired: 2 in, 2 out]
              n222 = Index Array(array=w219, index=2) -> (element=→"可能性":i32)
            }
            n223 = call <vilib>:"DAQmx Clear Task.vi"("task in"=w167, "error in"=w166) -> ("error out"=w165:errorcluster)  [unwired: 13 in]
            n224 = property on="start" class="Bool"(error in=w165, "DisabledEnum"=T2."Enabled" ("禁用")) -> (error out=w178:errorcluster)  [unwired: 1 in, 1 out]
            n225 = property on="stop" class="Bool"(error in=w178, "DisabledEnum"=T2."Disabled and Grayed Out" ("禁用")) -> (error out=w179:errorcluster)  [unwired: 1 in, 1 out]
            n226 = property on="save" class="Bool"(error in=w179, "DisabledEnum"=w149) -> (error out=w146:errorcluster)  [unwired: 1 in, 1 out]
            n227 = property on="Resistance" class="DigNum (严格)"(error in=w146, "DisabledEnum"=w149) -> (error out=w145:errorcluster)  [unwired: 1 in, 1 out]
            n228 = property on="close" class="Bool"(error in=w145, "DisabledEnum"=w149) -> (error out=w171:errorcluster)  [unwired: 1 in, 1 out]
            n229 = property on="Voltage" class="DigNum (严格)"(error in=w171, "DisabledEnum"=w149) -> (error out=w168:errorcluster)  [unwired: 1 in, 1 out]
            n230 = call "DAQ助手2"("data"=0.0 ("dt"), "error in"=w168) -> ()  [unwired: 16 in, 2 out]
          }
        }
      }
      frame #1 {
        n231 = case shown="真" "?" {
          tunnel: w360 -> [_ _]
          tunnel: w359 -> [_ _]
          tunnel: w360 -> [_ w364]
          tunnel: w359 -> [_ w363]
          frame False {
          }
          frame True {
            n232 = node(w364, w363, "creatdata", 0.0) -> ()  [unwired: 2 in, 4 out]
          }
        }
        n233 = case shown="真" "确定按钮 2" {
          frame False {
          }
          frame True {
            n234 = Current VI's Path() -> (path=w383:path)
            n235 = property class="App"() -> ("App.Kind"=w384:T3)  [unwired: 2 in, 2 out]
            n236 = Strip Path(path=w383) -> (stripped path=w385:path)  [unwired: 1 out]
            n237 = case shown="\"Development System\"" w384 {
              tunnel: w385 -> [w389 w390 w391 w392 w393 w394 w396]
              tunnel: [w389 w390 w391 w392 w393 w394 w395] -> w380
              frame "Development System" {
              }
              frame "Embedded LabVIEW" {
              }
              frame "Student Edition" {
              }
              frame "invalid app kind" {
              }
              frame "Custom" {
              }
              frame "Evaluation" {
              }
              frame "Run Time System" {
                n238 = Strip Path(path=w396) -> (stripped path=w395:path)  [unwired: 1 out]
              }
            }
            n239 = Build Path(base path=w380, name or relative path="train") -> (appended path=w379:path)
            n240 = Get Date/Time In Seconds() -> (seconds since 1Jan1904=w373:timestamp)
            n241 = Format Date/Time String(time format string (%c)="%H%M", seconds (now)=w373) -> (date/time string=w371:string)  [unwired: 1 in]
            n242 = Build Path(base path=w379, name or relative path="label") -> (appended path=w370:path)
            n243 = call <vilib>:"Check if File or Folder Exists.vi"("path"=w370) -> ("file or folder exists?"=w369:bool, "dup path"=w367:path)  [unwired: 8 in, 1 out]
            n244 = Concatenate Strings(w371, ".txt") -> (w377:string)
            n245 = case shown="假" w369 {
              tunnel: [w386 w388] -> w368
              tunnel: w367 -> [w387 w388]
              frame False {
                n246 = Create Folder(path (use dialog)=w387) -> (created path=w386:path)  [unwired: 2 in, 2 out]
              }
              frame True {
              }
            }
            n247 = Build Path(base path=w368, name or relative path=w377) -> (appended path=w374:path)
            n248 = property on="default" class="Path"() -> ("Value"=w376:path)  [unwired: 2 in, 2 out]
            n249 = Copy(9:TRUE ("覆盖(F)"), 10:w374, 11:w376) -> ()  [unwired: 2 in, 3 out]
          }
        }
      }
    }
    n250 = case shown="假" FALSE {
      frame False {
      }
      frame True {
        n251 = Current VI's Path() -> (path=w72:path)
        n252 = Open VI Reference(vi path=w72) -> (vi reference=w71:refnum<vi>)  [unwired: 5 in, 1 out]
        n253 = invoke class="VI" method="FP.Close"(reference=w71) -> ()  [unwired: 2 in, 3 out]
      }
    }
  }
